vi "Override Interpolation.vi"(0 "gen in":refnum<class "niUSRP Tx DSP v2 FPGA.lvclass">, 5 "interpolation with registers":refnum<class "Interpolation with Registers (IQ 18-bit).lvclass">) -> (4 "gen out":refnum<class "niUSRP Tx DSP v2 FPGA.lvclass">)   [LabVIEW 2025, in "niUSRP Tx DSP v2 FPGA.lvclass"]
uses:
  niUSRP Tx DSP v2 FPGA.lvclass
  <instrlib>/_niInstr/DSP Control/Common/v2/FPGA/Interpolation/IQ 18-bit with Regs/Interpolation with Registers (IQ 18-bit).lvclass
  C:/Program Files/NI/LVAddons/niidl/1/instr.lib/_niInstr/DSP Control/Interface/v1/FPGA/Interpolation/IQ 18-bit/Interpolation Interface (IQ 18-bit).lvclass
  <instrlib>/_niInstr/DSP Control/Interface/v1/FPGA/Interpolation/IQ 18-bit/Interpolation Interface (IQ 18-bit).lvclass
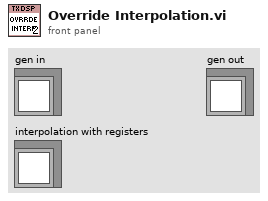
[diagram p1: front panel]
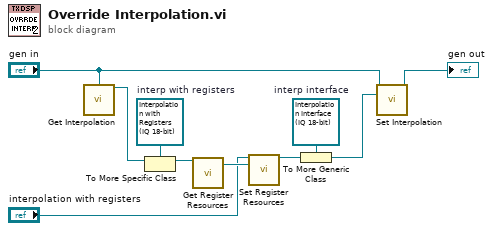
[diagram p0: block diagram]
diagram:
  w5 = refnum<class "Interpolation with Registers (IQ 18-bit).lvclass"> refnum  # interp with registers
  w7 = refnum<class "Interpolation Interface (IQ 18-bit).lvclass"> refnum  # interp interface
  n1 = call-dynamic "Get Interpolation.vi"("gen"="gen in") -> ("interpolation"=w1:refnum<class "Interpolation Interface (IQ 18-bit).lvclass">)  [unwired: 14 in]
  n2 = To More Specific Class(target class=w5, reference=w1) -> (specific class reference=w10:refnum<class "Interpolation with Registers (IQ 18-bit).lvclass">)  [unwired: 1 in, 1 out]
  n3 = call <instrlib>:"Get Register Resources.vi"("interpolation in"=w10) -> ("interpolation regs"=w6:refnum<class "Interpolation Registers.lvclass">)  [unwired: 13 in, 1 out]
  n4 = call <instrlib>:"Set Register Resources.vi"("interpolation in"="interpolation with registers", "interpolation regs"=w6) -> ("interpolation out"=w9:refnum<class "Interpolation with Registers (IQ 18-bit).lvclass">)  [unwired: 13 in]
  n5 = To More Generic Class(target class=w7, reference=w9) -> (generic class reference=w8:refnum<class "Interpolation Interface (IQ 18-bit).lvclass">)
  n6 = call-dynamic "Set Interpolation.vi"("gen in"="gen in", "interpolation"=w8) -> ("gen out"=→"gen out":refnum<class "niUSRP Tx DSP v2 FPGA.lvclass">)  [unwired: 13 in]
